vi "Speed Position (SubVI).vi"(9 "Speed":i16, 10 "Position":i16(knob) max=1023 scale=0.0..4096.0, 11 "ID":u8) -> (3 "result string":string)   [LabVIEW 2017]
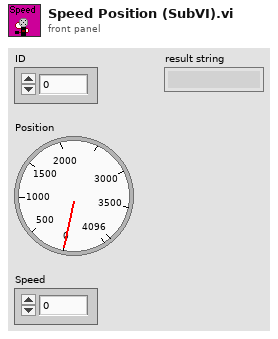
[diagram p1: front panel]
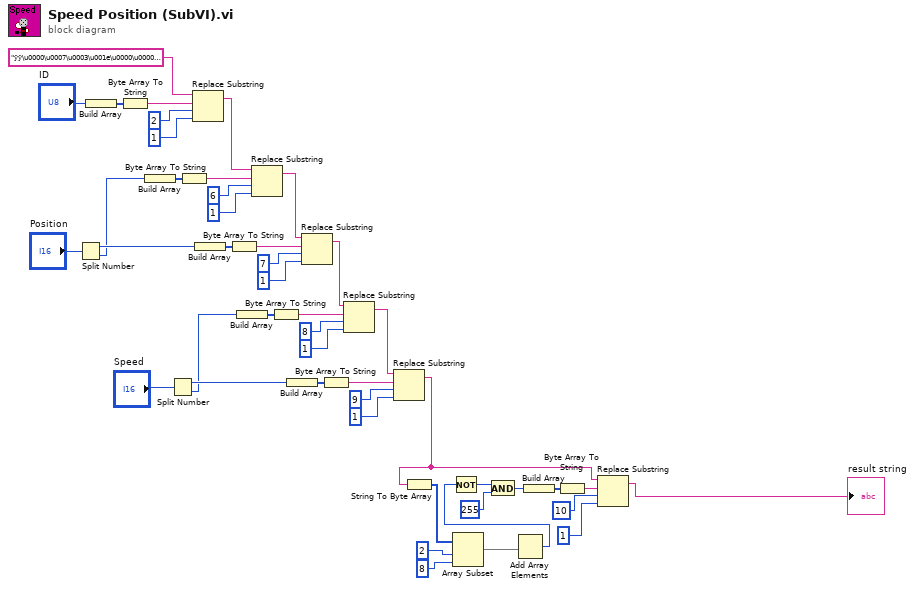
[diagram p0: block diagram]
diagram:
  n1 = Split Number(x="Position") -> (hi(x)=w2:u8, lo(x)=w1:u8)
  n2 = Build Array("ID") -> (w12:u8[])
  n3 = Byte Array To String(unsigned byte array=w12) -> (string=w10:string)
  n4 = Build Array(w1) -> (w16:u8[])
  n5 = Split Number(x="Speed") -> (hi(x)=w33:u8, lo(x)=w32:u8)
  n6 = Byte Array To String(unsigned byte array=w16) -> (string=w15:string)
  n7 = Replace Substring(2:1 ("length (len. of substring)"), 3:2 ("offset (0)"), 4:w10, 5:"ÿÿ\u0000\u0007\u0003\u001e\u0000\u0000\u0000\u0000\u0000" ("string")) -> (1:w19:string)  [unwired: 1 out]
  n8 = Build Array(w2) -> (w5:u8[])
  n9 = Byte Array To String(unsigned byte array=w5) -> (string=w4:string)
  n10 = Build Array(w32) -> (w40:u8[])
  n11 = Replace Substring(2:1 ("length (len. of substring)"), 3:6 ("offset (0)"), 4:w15, 5:w19) -> (1:w3:string)  [unwired: 1 out]
  n12 = Byte Array To String(unsigned byte array=w40) -> (string=w39:string)
  n13 = Build Array(w33) -> (w36:u8[])
  n14 = Replace Substring(2:1 ("length (len. of substring)"), 3:7 ("offset (0)"), 4:w4, 5:w3) -> (1:w43:string)  [unwired: 1 out]
  n15 = Byte Array To String(unsigned byte array=w36) -> (string=w35:string)
  n16 = Replace Substring(2:1 ("length (len. of substring)"), 3:8 ("offset (0)"), 4:w39, 5:w43) -> (1:w34:string)  [unwired: 1 out]
  n17 = Replace Substring(2:1 ("length (len. of substring)"), 3:9 ("offset (0)"), 4:w35, 5:w34) -> (1:w44:string)  [unwired: 1 out]
  n18 = String To Byte Array(string=w44) -> (unsigned byte array=w27:u8[])
  n19 = Array Subset(array=w27, index=2, length=8) -> (w30:u8[])
  n20 = Add Array Elements(numeric array=w30) -> (sum=w31:u8)
  n21 = Not(x=w31) -> (.not. x?=w20:u8)
  n22 = And(x=w20, y=u8 255) -> (x .and. y?=w26:u8)
  n23 = Build Array(w26) -> (w23:u8[])
  n24 = Byte Array To String(unsigned byte array=w23) -> (string=w22:string)
  n25 = Replace Substring(2:1 ("length (len. of substring)"), 3:10 ("offset (0)"), 4:w22, 5:w44) -> (1:→"result string":string)  [unwired: 1 out]
